vi "LOER_GetHelp.vi"(0 "XRef":T17, 1 "Point":T16, 2 "State In":T14={"Inputs"=1, "SelectedIndex"=0, "ClassInfo"=[], "Width"=120, "EventReg Type"=variant}) -> (14 "Standard Help Info":T12, 15 "Detailed Help Info":T9, 16 "Subitem Help Info":T3, 17 "Use Detailed Help?":T2, 18 "Use Subitem Help?":T2, 19 "Fatal Error Out":T1)   [LabVIEW 2016, in "LV Object Event Registration Node.xnode"]
uses:
  LV Object Event Registration Node.xnode
  <vilib>/XNodeSupport/XNodeXNodeRef.ctl
  <vilib>/XNodeSupport/XNodePoint.ctl
  <vilib>/XNodeSupport/XNodeInt.ctl
  LOER_State.ctl
  LOER_ClassInfo.ctl
  <vilib>/XNodeSupport/XNodeStandardHelpInfo.ctl
  <vilib>/XNodeSupport/XNodeString.ctl
  <vilib>/XNodeSupport/XNodePath.ctl
  <vilib>/XNodeSupport/XNodeDetailedHelpInfo.ctl
  <vilib>/XNodeSupport/XNodeImage.ctl
  <vilib>/XNodeSupport/XNodeRect32.ctl
  <vilib>/XNodeSupport/XNodeTerms.ctl
  <vilib>/XNodeSupport/XNodeTerm.ctl
  <vilib>/XNodeSupport/XNodeVariant.ctl
  <vilib>/XNodeSupport/XNodeBool.ctl
  <vilib>/XNodeSupport/XNodeSubitemHelpInfo.ctl
  <vilib>/XNodeSupport/XNodeErrorCluster.ctl
  <vilib>/XNodeSupport/NI_XNodeSupport.lvlib
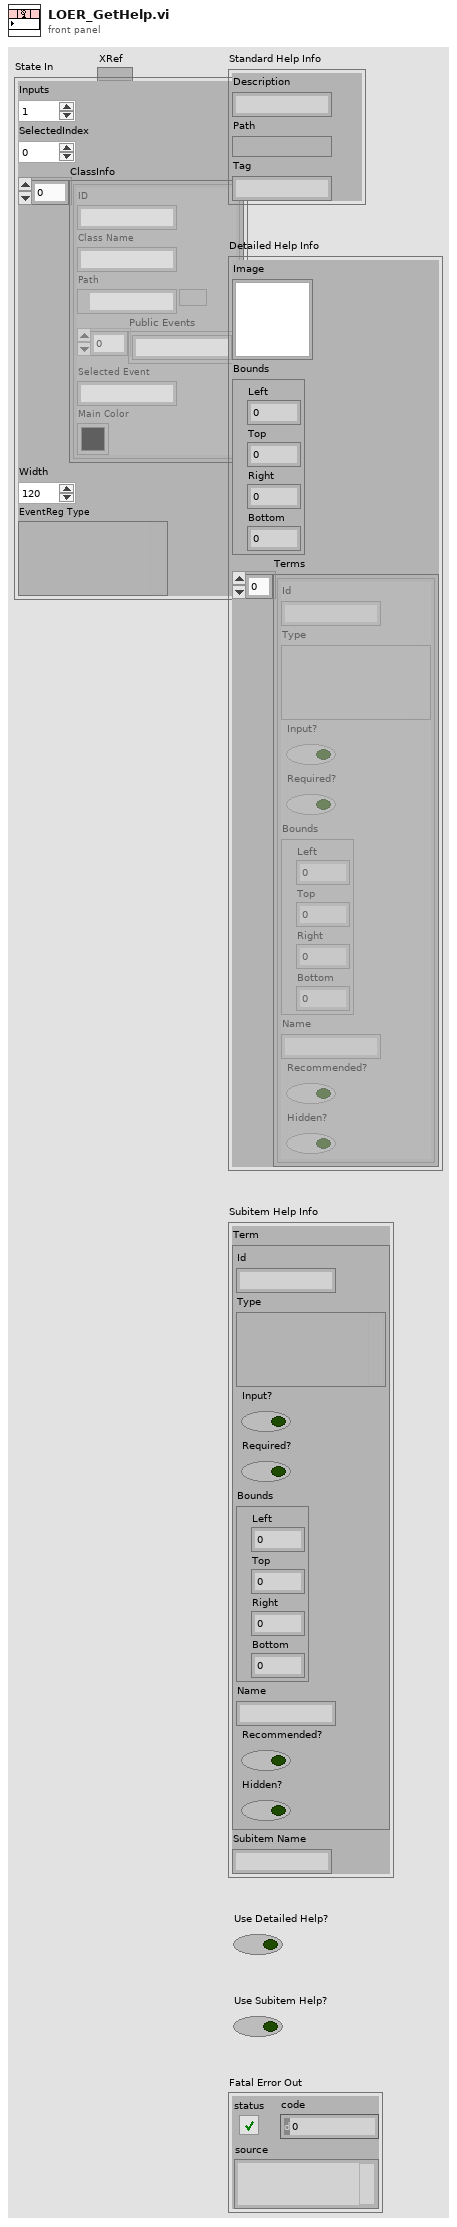
[diagram p1: front panel]
types:
  T1 = typedef "NI_XNodeSupport.lvlib/XNodeErrorCluster.ctl" = errorcluster
  T2 = typedef "NI_XNodeSupport.lvlib/XNodeBool.ctl" = bool
  T3 = typedef "NI_XNodeSupport.lvlib/XNodeSubitemHelpInfo.ctl" = cluster{"Term":T4, "Subitem Name":T5}
  T4 = typedef "NI_XNodeSupport.lvlib/XNodeTerm.ctl" = cluster{"Id":T5, "Type":T6, "Input?":T2, "Required?":T2, "Bounds":T7, "Name":T5, "Recommended?":T2, "Hidden?":T2}
  T5 = typedef "NI_XNodeSupport.lvlib/XNodeString.ctl" = string
  T6 = typedef "NI_XNodeSupport.lvlib/XNodeVariant.ctl" = variant
  T7 = typedef "NI_XNodeSupport.lvlib/XNodeRect32.ctl" = cluster{"Left":T8, "Top":T8, "Right":T8, "Bottom":T8}
  T8 = typedef "NI_XNodeSupport.lvlib/XNodeInt.ctl" = i32
  T9 = typedef "NI_XNodeSupport.lvlib/XNodeDetailedHelpInfo.ctl" = cluster{"Image":T10, "Bounds":T7, "Terms":T11}
  T10 = typedef "NI_XNodeSupport.lvlib/XNodeImage.ctl" = picture
  T11 = typedef "NI_XNodeSupport.lvlib/XNodeTerms.ctl" = T4[]
  T12 = typedef "NI_XNodeSupport.lvlib/XNodeStandardHelpInfo.ctl" = cluster{"Description":T5, "Path":T13, "Tag":T5}
  T13 = typedef "NI_XNodeSupport.lvlib/XNodePath.ctl" = path
  T14 = typedef "LV Object Event Registration Node.xnode/LOER_State.ctl" = cluster{"Inputs":u16, "SelectedIndex":i16, "ClassInfo":T15[], "Width":u16, "EventReg Type":variant}
  T15 = typedef "LV Object Event Registration Node.xnode/LOER_ClassInfo.ctl" = cluster{"ID":string, "Class Name":string, "Path":path, "Public Events":string[], "Selected Event":string, "Main Color":u32}
  T16 = typedef "NI_XNodeSupport.lvlib/XNodePoint.ctl" = cluster{"H":T8, "V":T8}
  T17 = typedef "NI_XNodeSupport.lvlib/XNodeXNodeRef.ctl" = refnum<vi>
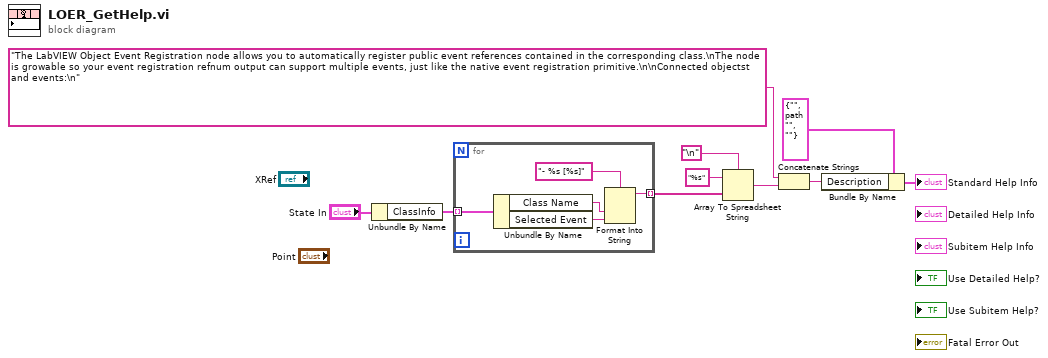
[diagram p0: block diagram]
diagram:
  n1 = Unbundle By Name("State In") -> ("ClassInfo"=w7:T15[])
  n2 = for {
    tunnel: w7 -> [w15] mode=indexing
    tunnel: [w11] -> w4 mode=indexing
    n3 = Unbundle By Name(w15) -> ("Class Name"=w13:string, "Selected Event"=w12:string)
    n4 = Format Into String(format string="- %s [%s]", w13, w12) -> (resulting string=w11:string)  [unwired: 2 in, 1 out]
  }
  n5 = Array To Spreadsheet String(delimiter (Tab)="\n", array=w4, 3:"%s" ("format string")) -> (spreadsheet string=w2:string)
  n6 = Concatenate Strings("The LabVIEW Object Event Registration node allows you to automatically register public event references contained in the corresponding class.\nThe node is growable so your event registration refnum output can support multiple events, just like the native event registration primitive.\n\nConnected objectst and events:\n" ("string"), w2) -> (w1:string)
  n7 = Bundle By Name(cluster=T12 {"Description"="", "Path"=path "", "Tag"=""} ("Standard Help Info"), "Description"=w1) -> (→"Standard Help Info":T12)
